vi "Subtree Hierarchy.vi"(8 "error in (no error)":errorcluster, 11 "Config Storage in":refnum<class "Config Storage.lvclass">) -> (0 "error out":errorcluster, 2 "Subtree Hierarchy":string[](array[string]), 3 "Config Storage out":refnum<class "Config Storage.lvclass">)   [LabVIEW 2020, in "CDM-Config.lvlib" / "Config Storage.lvclass"]
uses:
  Config Storage.lvclass
  Config Storage.lvclass/Config Storage.ctl
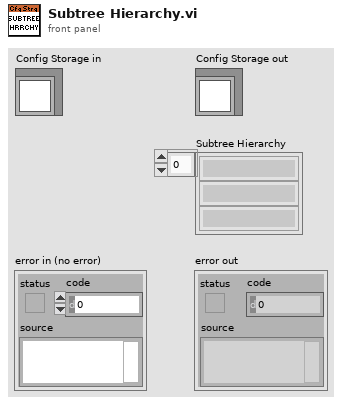
[diagram p1: front panel]
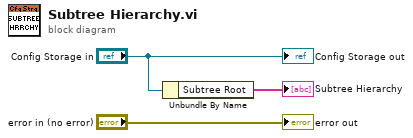
[diagram p0: block diagram]
diagram:
  n1 = Unbundle By Name("Config Storage in") -> ("Subtree Root"=→"Subtree Hierarchy":string[])
  "error out" <- "error in (no error)"
  "Config Storage out" <- "Config Storage in"
